vi "Seconds since 1904 Months ago.vi"(1 "No of Months ago":i32) -> (0 "Seconds since 1904":dbl format="%#.0f")   [LabVIEW 2022 SP3]
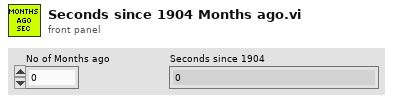
[diagram p1: front panel]
types:
  T1 = typedef "LVDateTimeRec.ctl" = cluster{"fractional second":dbl, "second":i32, "minute":i32, "hour":i32, "day of month":i32, "month":i32, "year":i32, "day of week":i32, "day of year":i32, "DST":i32}
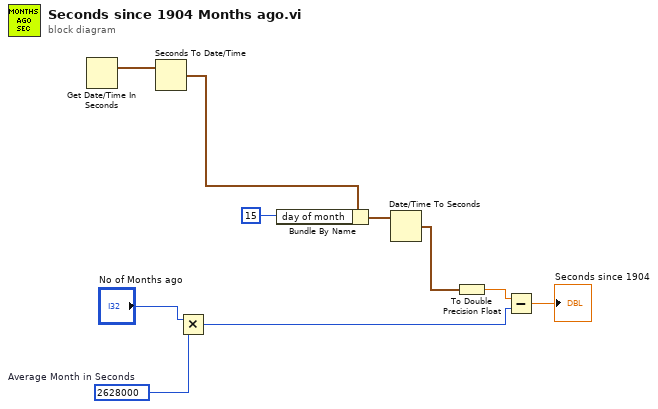
[diagram p0: block diagram]
diagram:
  w5 = 2628000  # Average Month in Seconds
  n1 = Get Date/Time In Seconds() -> (seconds since 1Jan1904=w10:timestamp)
  n2 = Seconds To Date/Time(time stamp (now)=w10) -> (date time rec=w9:T1)  [unwired: 1 in]
  n3 = Multiply(x="No of Months ago", y=w5) -> (x*y=w2:i32)
  n4 = Bundle By Name(cluster=w9, "day of month"=15) -> (w7:T1)
  n5 = Date/Time To Seconds(2:w7) -> (0:w4:timestamp)  [unwired: 1 in]
  n6 = To Double Precision Float(number=w4) -> (double precision float=w3:dbl)
  n7 = Subtract(x=w3, y=w2) -> (x-y=→"Seconds since 1904":dbl)
